vi "Actor Core.vi"(8 "error in":errorcluster, 11 "Nested in":refnum<class "User Inteface.lvclass">) -> (0 "error out":errorcluster, 3 "Actor out":refnum<class "Actor.lvclass">)   [LabVIEW 2020, in "User Inteface.lvlib" / "User Inteface.lvclass"]
doc: "(<B>Filename</B>: Actor Framework.lvlib:Actor.lvclass:Actor Core.vi)\n\nReceives messages to the actor, reacts to them, and initiates any error handling that may shut the actor down.\n\nDescendant classes may override this VI to append parallel tasks for the actor to complete while it handles messages. Overrides use the Call Parent Method node."
uses:
  User Inteface.lvclass
  C:/Program Files (x86)/National Instruments/LabVIEW 2020/vi.lib/ActorFramework/Actor/Actor.lvclass
  <vilib>/ActorFramework/Actor/Actor.lvclass
  No UI/No UI/No UI.lvclass
  <vilib>/ActorFramework/Actor/Actor.lvclass/Actor.ctl
  <vilib>/ActorFramework/Message Enqueuer/Message Enqueuer.lvclass/Message Enqueuer.ctl
  User Inteface.lvclass/User Inteface.ctl
  Si UI/Si UI.lvclass
  Si UI/Si UI.lvclass/Si UI.ctl
  <vilib>/ActorFramework/Message Enqueuer/Init from Existing Queue.vi
  <vilib>/ActorFramework/Message Enqueuer/Enqueue.vi
  <vilib>/ActorFramework/Stop Msg/Stop Msg.lvclass
  C:/Program Files (x86)/National Instruments/LabVIEW 2020/vi.lib/ActorFramework/Message/Message.lvclass
  <vilib>/ActorFramework/Message Priority Queue/Priority Enqueue.vi
  <vilib>/ActorFramework/Message Enqueuer/Message Enqueuer.lvclass
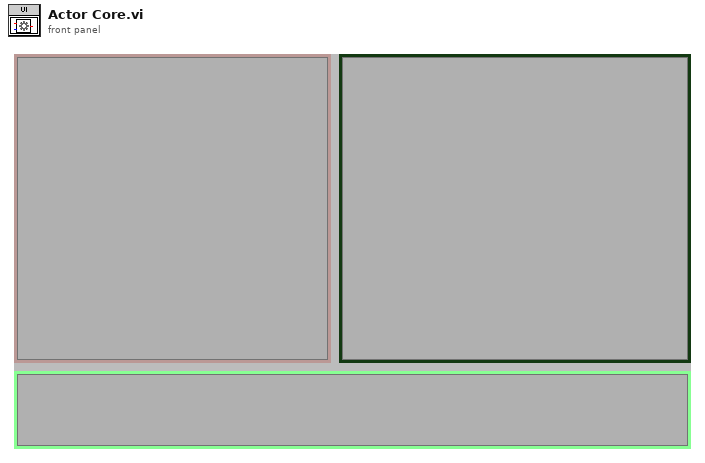
[diagram p1: front panel]
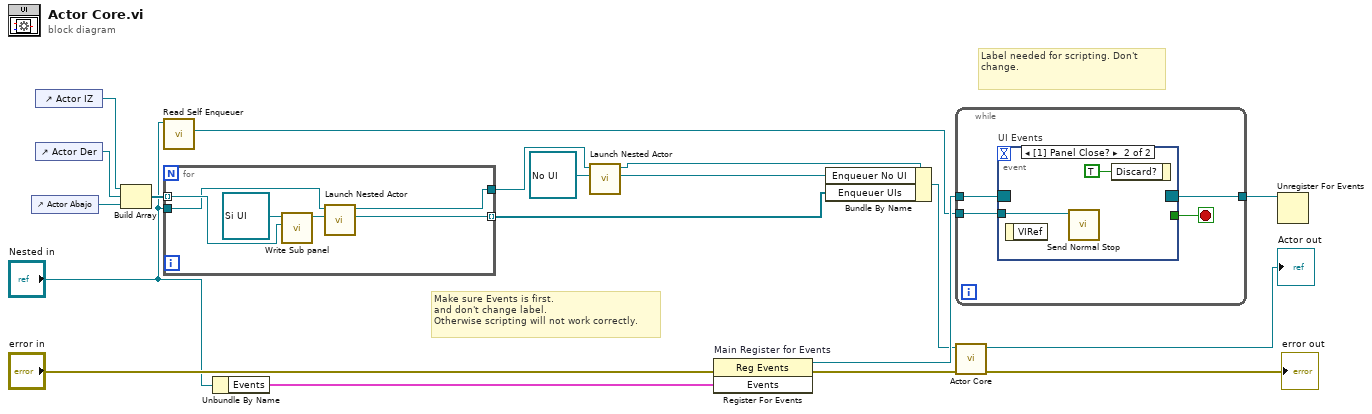
[diagram p0: block diagram]
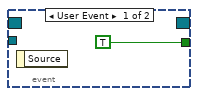
[diagram p2: hidden frame]
diagram:
  # "Label needed for scripting. Don't change."
  # "Make sure Events is first.\nand don't change label.\nOtherwise scripting will not work correctly."
  n1 = control-ref of="Actor Abajo"() -> (w6:refnum<vi>)
  n2 = control-ref of="Actor IZ"() -> (w8:refnum<vi>)
  n3 = control-ref of="Actor Der"() -> (w7:refnum<vi>)
  n4 = Build Array(w8, w7, w6) -> (w5:refnum<vi>[])
  n5 = call <vilib>:"Read Self Enqueuer.vi"("Actor"="Nested in") -> ("Self Enqueuer"=w14:refnum<class "Message Enqueuer.lvclass">)  [unwired: 10 in]
  n6 = for {
    tunnel: [w25] -> w10 mode=indexing
    tunnel: w5 -> [w23] mode=indexing
    tunnel: "Nested in" -> [w21]
    tunnel: [w20] -> w2
    n7 = call "Write Sub panel.vi"("Sub panel"=w23, "Si UI in"=refnum<class "Si UI.lvclass"> refnum ("Si UI.lvlib:Si UI.lvclass")) -> ("Si UI out"=w22:refnum<class "Si UI.lvclass">)  [unwired: 9 in]
    n8 = call <vilib>:"Launch Nested Actor.vi"("Nested Actor"=w22, "Caller Actor in"=w21) -> ("Nested Actor's Enqueuer"=w25:refnum<class "Message Enqueuer.lvclass">, "Caller Actor out"=w20:refnum<class "User Inteface.lvclass">)  [unwired: 7 in, 1 out]
  }
  n9 = Unbundle By Name("Nested in") -> ("Events"=w16:cluster{"Stop":refnum<user-event>})
  n10 = call <vilib>:"Launch Nested Actor.vi"("Nested Actor"=refnum<class "No UI.lvclass"> refnum ("No UI.lvlib:No UI.lvclass"), "Caller Actor in"=w2) -> ("Nested Actor's Enqueuer"=w9:refnum<class "Message Enqueuer.lvclass">, "Caller Actor out"=w1:refnum<class "User Inteface.lvclass">)  [unwired: 7 in, 1 out]
  n11 = register-events "Main Register for Events"(error in="error in", w16) -> (reference out=w17:refnum<event-registration>, error out=w12:errorcluster)  [unwired: 1 in]
  n12 = Bundle By Name(cluster=w1, "Enqueuer No UI"=w9, "Enqueuer UIs"=w10) -> (w11:refnum<class "User Inteface.lvclass">)
  n13 = while {
    tunnel: w17 -> [w29]
    tunnel: [w27] -> w15
    tunnel: w14 -> [w26]
    stop <- w28 stop-if-true
    n14 = event "UI Events" shown="[1] Panel Close?" {
      selector: w29 -> [_ _]
      dyn-events: [_ _] -> w27
      timeout: _ -> [_ _]
      tunnel: [TRUE _] -> w28
      tunnel: w26 -> [_ w31]
      event User Event {
        n15 = event-data() -> ()  [unwired: 1 in, 1 out]
      }
      event Panel Close? {
        n16 = event-data() -> ()  [unwired: 1 in, 1 out]
        n17 = call <vilib>:"Send Normal Stop.vi"("Message Enqueuer"=w31) -> ()  [unwired: 10 in, 1 out]
        n18 = event-data("Discard?"=TRUE) -> ()  [unwired: 1 in, 1 out]
      }
    }
  }
  n19 = call-parent "Actor Core.vi"("error in"=w12, "Actor in"=w11) -> ("error out"=→"error out":errorcluster, "Actor out"=→"Actor out":refnum<class "Actor.lvclass">)  [unwired: 8 in]
  n20 = Unregister For Events(event registration refnum=w15) -> ()  [unwired: 1 in, 1 out]
